vi "Get Variant Message.vi"(8 "error in (no error)":errorcluster, 11 "Message Double in":refnum<class "Message 2D String Array.lvclass">) -> (0 "error out":errorcluster, 1 "Value":variant, 2 "Name":string, 3 "Message Double out":refnum<class "Message 2D String Array.lvclass">)   [LabVIEW 2016, in "WebSocket Networking.lvlib" / "Message 2D String Array.lvclass"]
doc: "--\nCopyright © 2017 Composed SystemsI All rights reserved.\n\nAuthor: Jon McBee <jon.mcbee@composed.io>\n\nThis library is provided \"AS IS\" ,WITHOUT WARRANTIES OR\nCONDITIONS OF ANY KIND, either express or implied.\n\nComposed Systems -- composed.io\n\nStream 0.0.1.1\nJon McBee - Composed Systems\nCopyright (c) 2017, Composed Systems"
uses:
  <userlib>/Common Components/WebSocket Networking/Message 2D String Array/Message 2D String Array.lvclass
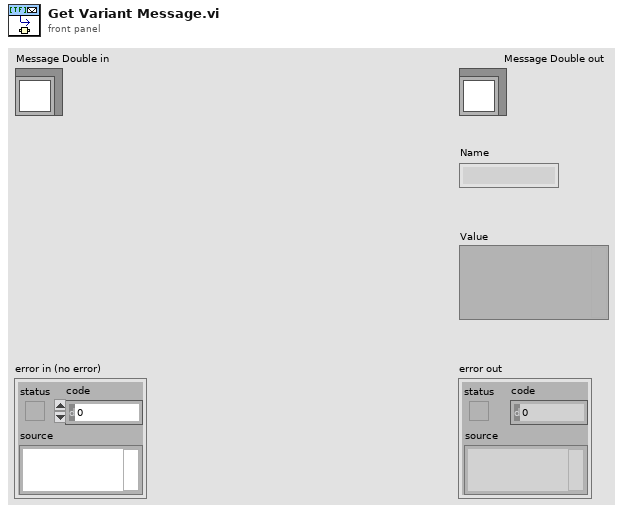
[diagram p1: front panel]
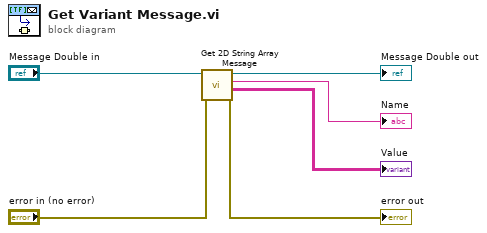
[diagram p0: block diagram]
diagram:
  n1 = call <userlib>:"Get 2D String Array Message.vi"("error in (no error)"="error in (no error)", "Message Double in"="Message Double in") -> ("error out"=→"error out":errorcluster, "Value"=→"Value":string[][], "Name"=→"Name":string, "Message Double out"=→"Message Double out":refnum<class "Message 2D String Array.lvclass">)  [unwired: 6 in]
